vi "CMN_testpath.vi"(8 "error in":errorcluster, 10 "ModuleName":string, 11 "caller Path":path) -> (0 "error out":errorcluster, 2 "ConfigFile":path)   [LabVIEW 2016]
panel:
  out "path":path
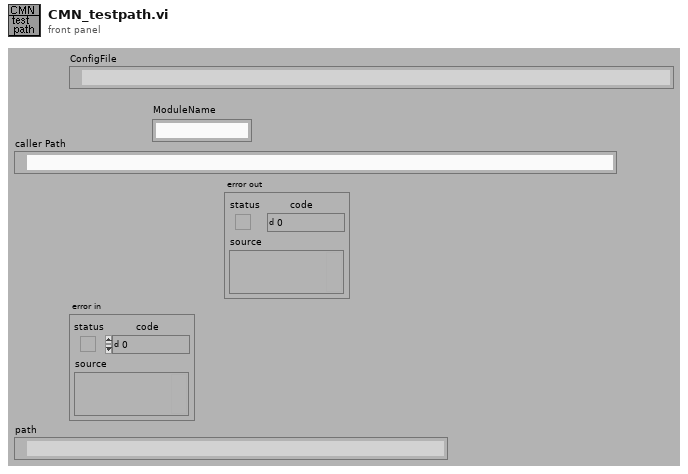
[diagram p1: front panel]
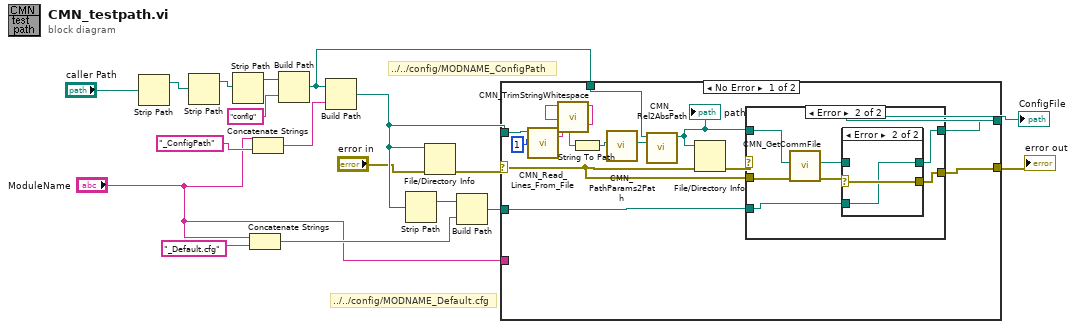
[diagram p0: block diagram]
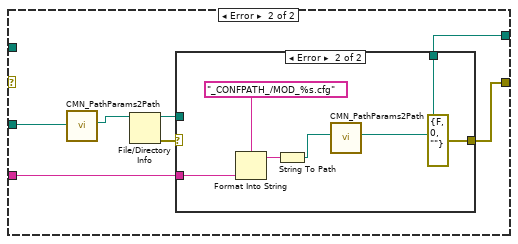
[diagram p4: hidden frame]
diagram:
  # "../../config/MODNAME_ConfigPath"
  # "../../config/MODNAME_Default.cfg"
  n1 = Strip Path(path="caller Path") -> (stripped path=w8:path)  [unwired: 1 out]
  n2 = Strip Path(path=w8) -> (stripped path=w7:path)  [unwired: 1 out]
  n3 = Strip Path(path=w7) -> (stripped path=w5:path)  [unwired: 1 out]
  n4 = Concatenate Strings("ModuleName", "_Default.cfg" ("string")) -> (w14:string)
  n5 = Concatenate Strings("ModuleName", "_ConfigPath" ("string")) -> (w6:string)
  n6 = Build Path(base path=w5, name or relative path="config") -> (appended path=w1:path)
  n7 = Build Path(base path=w1, name or relative path=w6) -> (appended path=w13:path)
  n8 = Strip Path(path=w13) -> (stripped path=w17:path)  [unwired: 1 out]
  n9 = File/Directory Info(path=w13, error in="error in") -> (error out=w18:errorcluster)  [unwired: 6 out]
  n10 = Build Path(base path=w17, name or relative path=w14) -> (appended path=w12:path)
  n11 = case shown="No Error" w18 {
    selector: w18 -> [w27 _]
    tunnel: w13 -> [w20 _]
    tunnel: [w30 w47] -> w3
    tunnel: w12 -> [w29 w51]
    tunnel: [w28 w49] -> w11
    tunnel: "ModuleName" -> [_ w46]
    tunnel: w1 -> [w19 _]
    frame No Error {
      n12 = call "CMN_Read_Lines_From_File.vi"("file path"=w20, "number of lines (all:-1)"=1) -> ("line string"=w25:string)  [unwired: 7 out]
      n13 = call "CMN_TrimStringWhitespace.vi"("string"=w25) -> ("trimmed string"=w24:string)  [unwired: 1 in, 8 out]
      n14 = String To Path(string=w24) -> (path=w23:path)
      n15 = call "CMN_PathParams2Path.vi"("Path In"=w23) -> ("Path out"=w22:path)  [unwired: 2 in, 8 out]
      n16 = call "CMN_Rel2AbsPath.vi"("test path"=w22, "absolute path"=w19) -> ("output path"=w21:path)  [unwired: 1 in, 8 out]
      "path" <- w21
      n17 = File/Directory Info(path=w21, error in=w27) -> (error out=w31:errorcluster)  [unwired: 6 out]
      n18 = case shown="Error" w31 {
        tunnel: w21 -> [w33 w40]
        tunnel: [w33 w38] -> w30
        tunnel: w29 -> [_ w35]
        tunnel: [w32 w36] -> w28
        tunnel: w27 -> [w32 w34]
        frame No Error {
        }
        frame Error {
          n19 = call "CMN_GetCommFile.vi"("error in (no error)"=w34, "path in"=w40) -> ("error out"=w39:errorcluster, "path out"=w37:path)  [unwired: 8 out]
          n20 = case shown="Error" w39 {
            selector: w39 -> [w41 w44]
            tunnel: [w42 w43] -> w38
            tunnel: w37 -> [w42 _]
            tunnel: [w41 w44] -> w36
            tunnel: w35 -> [_ w43]
            frame No Error {
            }
            frame Error {
            }
          }
        }
      }
    }
    frame Error {
      n21 = call "CMN_PathParams2Path.vi"("Path In"=w51) -> ("Path out"=w45:path)  [unwired: 2 in, 8 out]
      n22 = File/Directory Info(path=w45) -> (path out=w48:path, error out=w50:errorcluster)  [unwired: 1 in, 5 out]
      n23 = case shown="Error" w50 {
        selector: w50 -> [w53 _]
        tunnel: [w53 errorcluster {"status"=FALSE, "code"=0, "source"=""} ("error IO")] -> w49
        tunnel: w48 -> [w52 _]
        tunnel: [w52 w55] -> w47
        tunnel: w46 -> [_ w59]
        frame No Error {
        }
        frame Error {
          n24 = Format Into String(format string="_CONFPATH_/MOD_%s.cfg", w59) -> (resulting string=w57:string)  [unwired: 2 in, 1 out]
          n25 = String To Path(string=w57) -> (path=w56:path)
          n26 = call "CMN_PathParams2Path.vi"("Path In"=w56) -> ("Path out"=w55:path)  [unwired: 2 in, 8 out]
        }
      }
    }
  }
  "error out" <- w11
  "ConfigFile" <- w3
